vi "OpenChekResTab.vi"   [LabVIEW 2023]
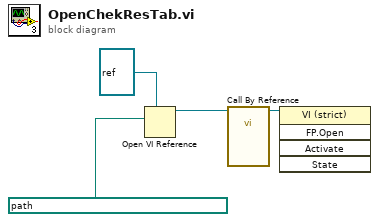
[diagram p0: block diagram]
diagram:
  n1 = Open VI Reference(type specifier VI Refnum (for type only)=refnum<vi> refnum, vi path=path "/Users/blagojnikolov/Library/Mobile Documents/com~apple~CloudDocs/» LabView/LabView/Project'24/Projects/649/subVI Tools/CollorCellsInTableOnly.vi") -> (vi reference=w2:refnum<vi>)  [unwired: 4 in, 1 out]
  n2 = call-by-ref "?"(reference=w2) -> (reference out=w1:refnum<vi>)  [unwired: 12 in, 2 out]
  n3 = invoke class="VI (strict)" method="FP.Open"(reference=w1) -> ()  [unwired: 4 in, 5 out]
